vi "Tray_WarnMsg.vi"(7 "SingleBtn":bool, 9 "Boolean Text Cancel":string, 10 "Boolean Text OK":string, 11 "Msg":string) -> (3 "OK?":bool)   [LabVIEW 2015]
uses:
  <vilib>/Utility/miscctls.llb/LVPointTypeDef.ctl
  <vilib>/Utility/miscctls.llb/LVPositionTypeDef.ctl
panel:
  in  "Btn_Canel":bool
  in  "Btn_OK":bool
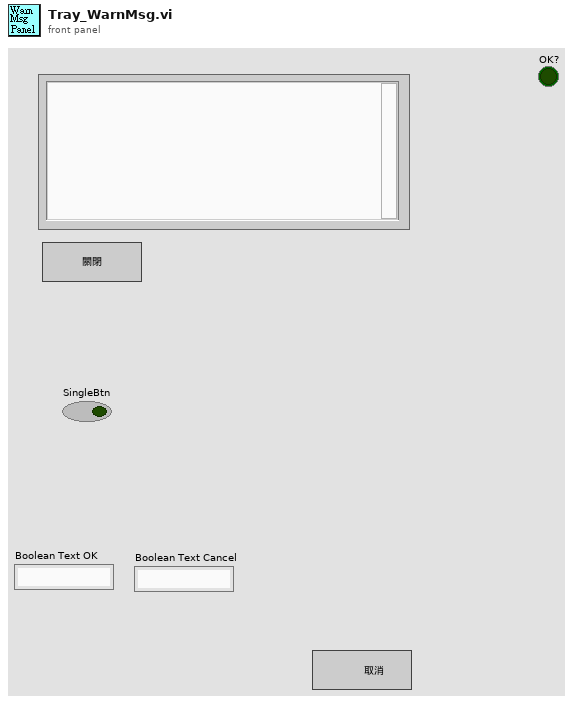
[diagram p1: front panel]
types:
  T1 = typedef "LVPointTypeDef.ctl" = cluster{"Horizontal":i16, "Vertical":i16}
  T2 = typedef "LVPositionTypeDef.ctl" = cluster{"Left":i32, "Top":i32}
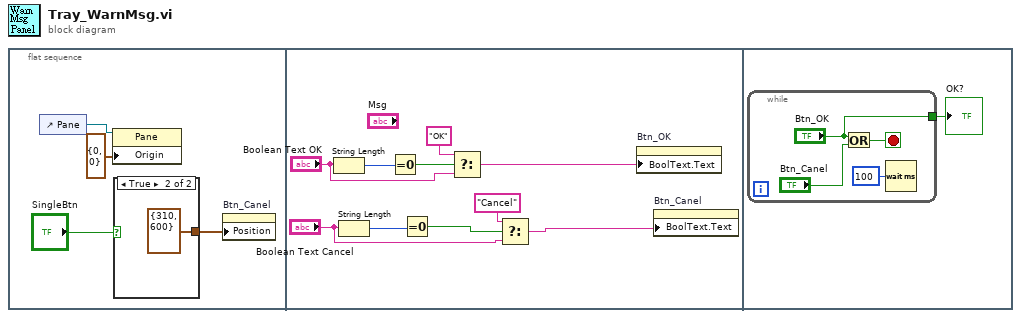
[diagram p0: block diagram]
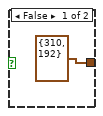
[diagram p2: hidden frame]
diagram:
  n1 = flat-sequence {
    frame #0 {
      n2 = control-ref of="Pane"() -> (w4:refnum<vi>)
      n3 = property class="Pane"(reference=w4, "Origin"=T1 {"Horizontal"=0, "Vertical"=0}) -> ()  [unwired: 1 in, 2 out]
      n4 = case shown="True" "SingleBtn" {
        tunnel: [T2 {"Left"=310, "Top"=192} ("Position") T2 {"Left"=310, "Top"=600} ("Position")] -> w2
        frame False {
        }
        frame True {
        }
      }
      n5 = property on="Btn_Canel" class="Bool"("Position"=w2) -> ()  [unwired: 2 in, 2 out]
    }
    frame #1 {
      n6 = String Length(string="Boolean Text OK") -> (length=w16:i32)
      n7 = String Length(string="Boolean Text Cancel") -> (length=w15:i32)
      n8 = Equal To 0?(x=w16) -> (x = 0?=w14:bool)
      n9 = Equal To 0?(x=w15) -> (x = 0?=w9:bool)
      n10 = Select(t="OK", s=w14, f="Boolean Text OK") -> (s? t:f=w11:string)
      n11 = Select(t="Cancel", s=w9, f="Boolean Text Cancel") -> (s? t:f=w7:string)
      n12 = property on="Btn_OK" class="Bool"("BoolText.Text"=w11) -> ()  [unwired: 2 in, 2 out]
      n13 = property on="Btn_Canel" class="Bool"("BoolText.Text"=w7) -> ()  [unwired: 2 in, 2 out]
    }
    frame #2 {
      n14 = while {
        tunnel: ["Btn_OK"] -> w17
        stop <- w20 stop-if-true
        n15 = Or(x="Btn_OK", y="Btn_Canel") -> (x .or. y?=w20:bool)
        n16 = Wait (ms)(milliseconds to wait=u32 100 ("millisecond timer value")) -> ()  [unwired: 1 out]
      }
      "OK?" <- w17
    }
  }
